vi "UHR-Fleezers Control (host) - 12.2.vi"() -> ()   [LabVIEW 2012] (continued)
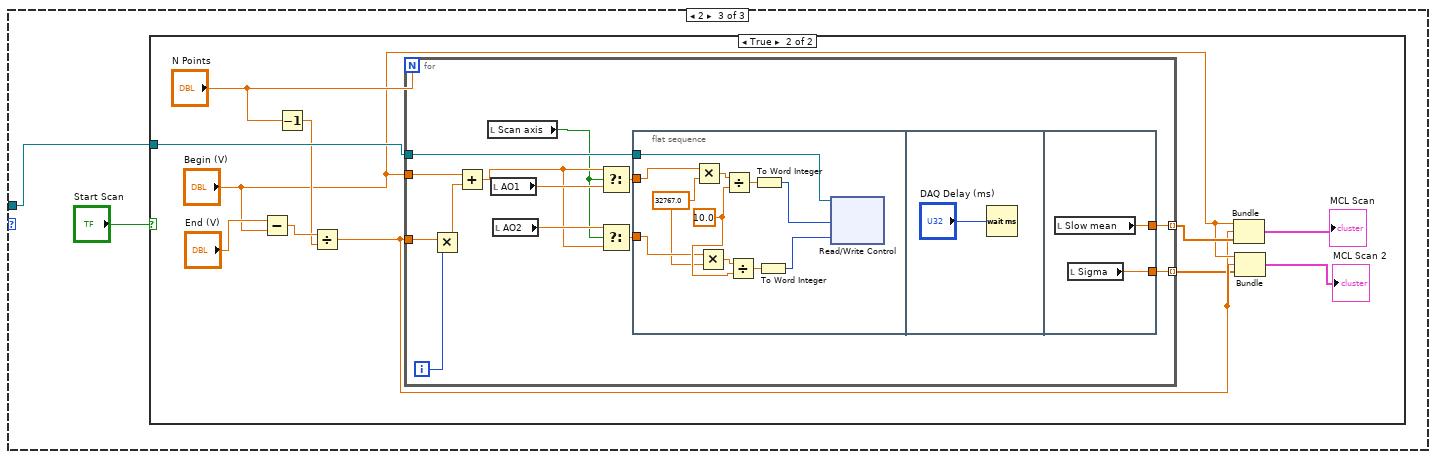
[diagram p3: hidden frame]
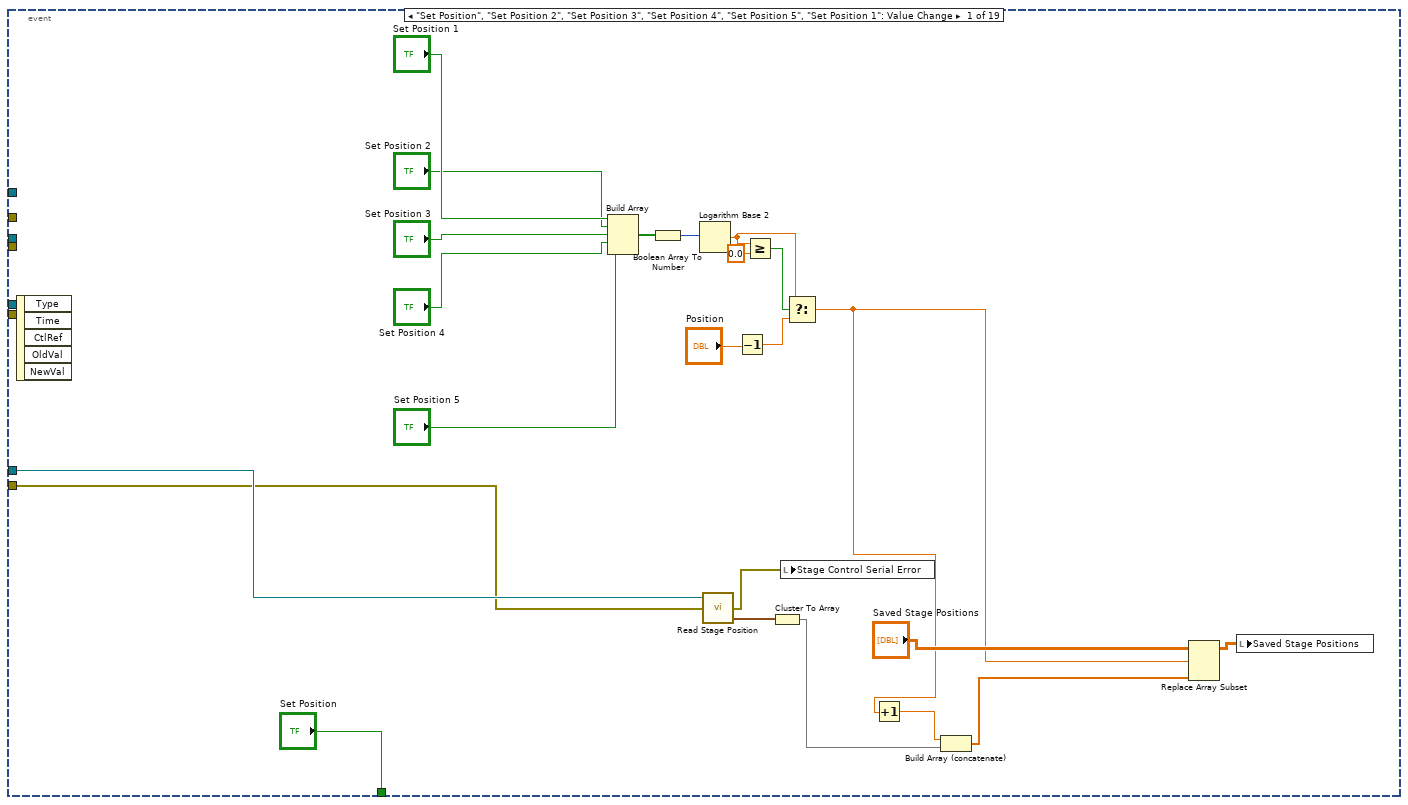
[diagram p6: hidden frame]
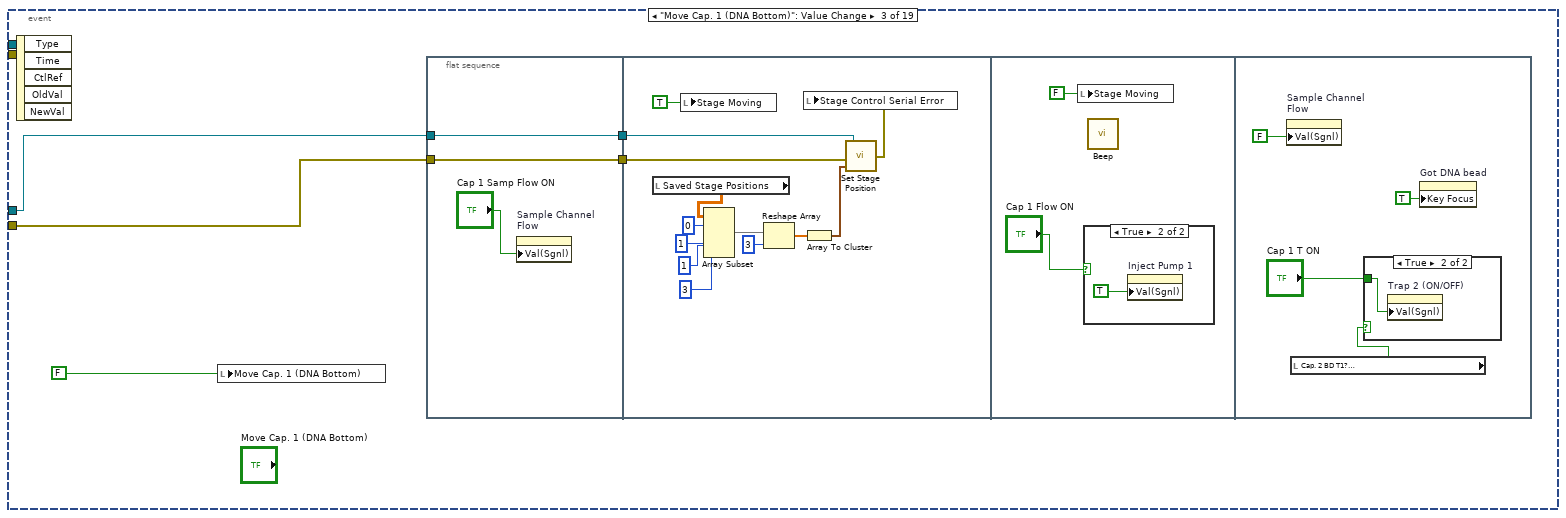
[diagram p7: hidden frame]
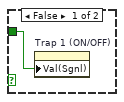
[diagram p9: hidden frame]
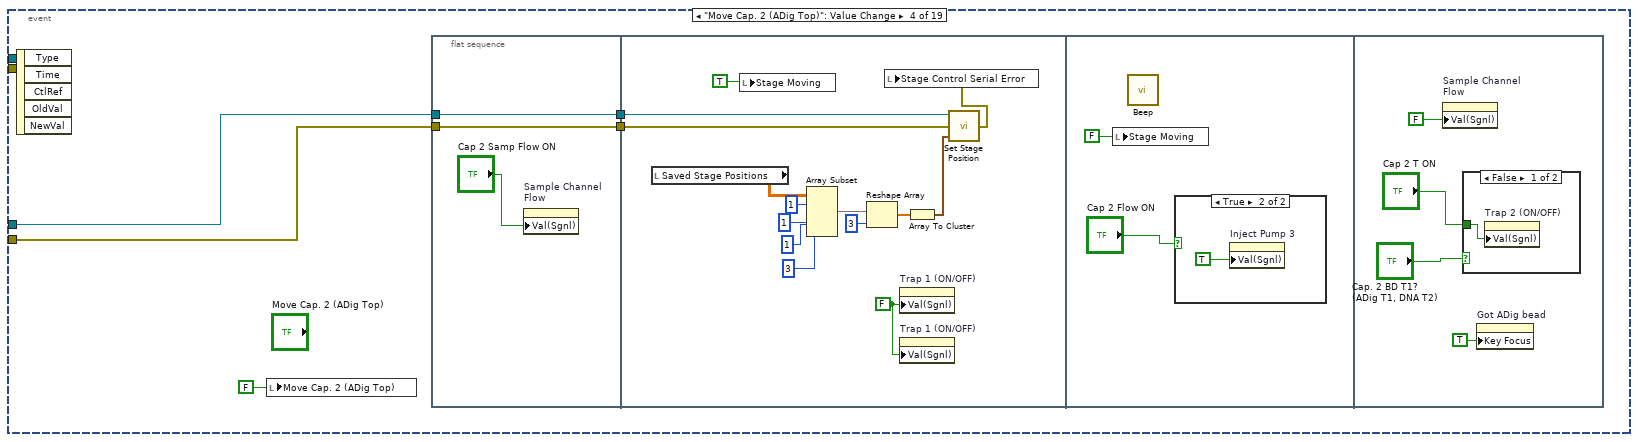
[diagram p10: hidden frame]
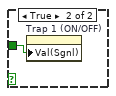
[diagram p12: hidden frame]
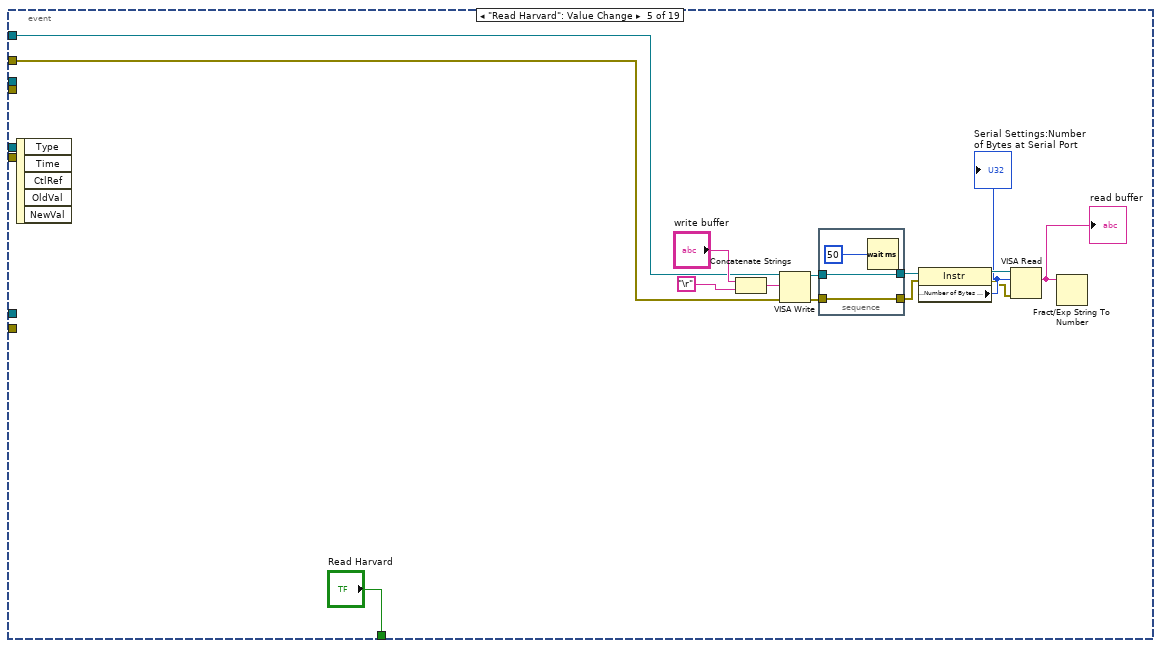
[diagram p13: hidden frame]
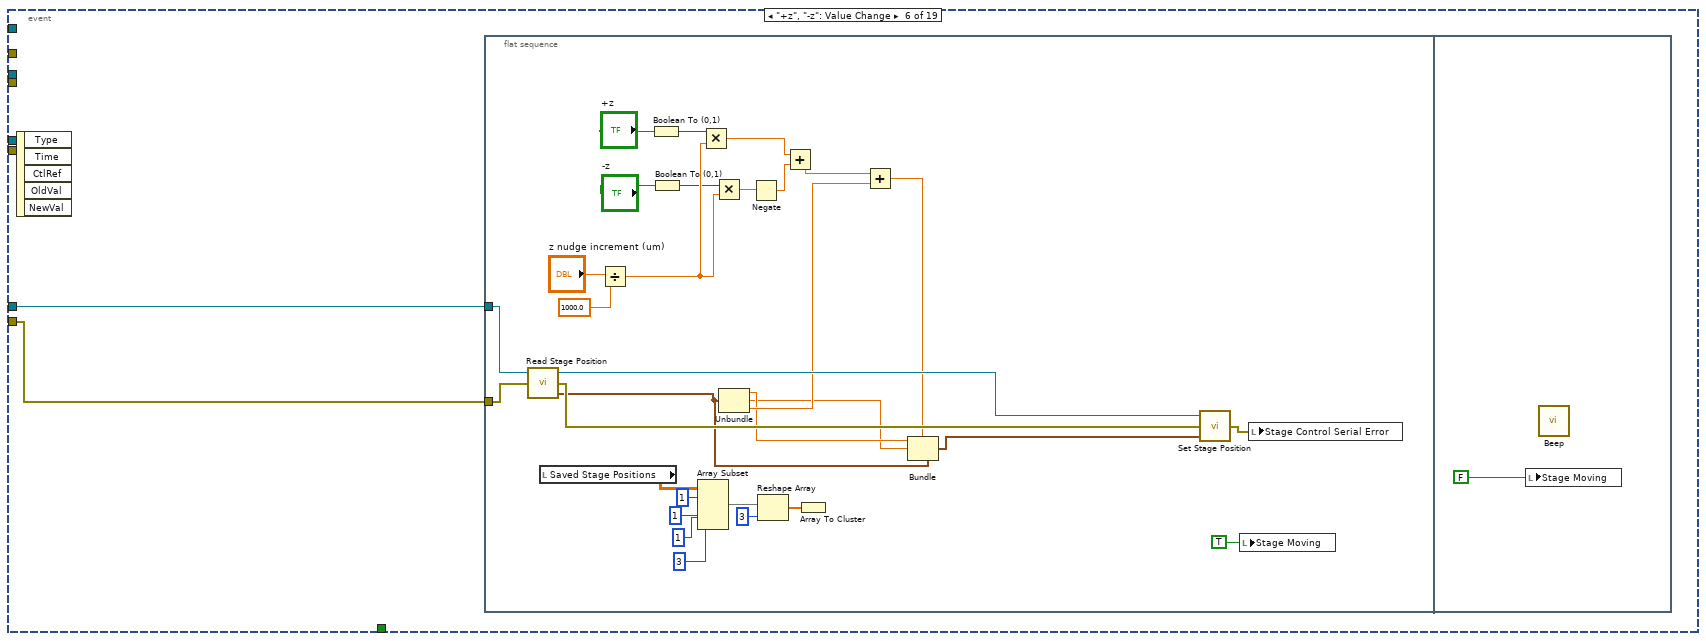
[diagram p14: hidden frame]
                                frame "Image", Default {
                                }
                                frame "Yank" {
                                n2869 = flat-sequence {
                                tunnel: [w4697] -> w4695
                                tunnel: w4694 -> [w4697]
                                tunnel: [w4696] -> w4693
                                tunnel: w4692 -> [w4696]
                                tunnel: w4695 -> [w4703]
                                tunnel: w4693 -> [w4701]
                                frame #0 {
                                n2870 = local read "Yank Delay (s)"() -> (w4700:dbl)
                                n2871 = Multiply(x=w4700, y=1000.0) -> (x*y=w4698:dbl)
                                n2872 = Wait (ms)(milliseconds to wait=w4698) -> ()  [unwired: 1 out]
                                }
                                frame #1 {
                                n2873 = local read "Yank to which?"() -> (w4702:bool)
                                n2874 = case shown="False" w4702 {
                                tunnel: w4703 -> [_ w4731]
                                tunnel: w4701 -> [w4704 _]
                                frame False {
                                n2875 = flat-sequence {
                                tunnel: w4704 -> [w4705]
                                frame #0 {
                                n2876 = property on="Trap Pos FB SP" class="DigNum (strict)"("Val(Sgnl)"=w4705) -> ()  [unwired: 2 in, 2 out]
                                }
                                frame #1 {
                                n2877 = Wait (ms)(milliseconds to wait=u32 700) -> ()  [unwired: 1 out]
                                }
                                frame #2 {
                                n2878 = local read "Action (%)"() -> (w4710:dbl)
                                n2879 = Absolute Value(x=w4710) -> (abs(x)=w4709:dbl)
                                n2880 = Greater?(x=w4709, y=70.0) -> (0:w4707:bool)
                                n2881 = property on="Remove Action Offset" class="Bool (strict)"("Val(Sgnl)"=w4707) -> ()  [unwired: 2 in, 2 out]
                                }
                                frame #3 {
                                n2882 = for {
                                N: 4 -> [_]
                                n2883 = flat-sequence {
                                frame #0 {
                                n2884 = Wait (ms)(milliseconds to wait=u32 500) -> ()  [unwired: 1 out]
                                }
                                frame #1 {
                                n2885 = local read "Action (%)"() -> (w4716:dbl)
                                n2886 = Absolute Value(x=w4716) -> (abs(x)=w4715:dbl)
                                n2887 = Greater?(x=w4715, y=70.0) -> (0:w4713:bool)
                                n2888 = property on="Remove Action Offset" class="Bool (strict)"("Val(Sgnl)"=w4713) -> ()  [unwired: 2 in, 2 out]
                                }
                                }
                                }
                                }
                                frame #4 {
                                n2889 = Wait (ms)(milliseconds to wait=u32 500) -> ()  [unwired: 1 out]
                                }
                                frame #5 {
                                n2890 = local read "Shift confocal"() -> (w4721:bool)
                                n2891 = local read "Mean"() -> (w4724:dbl)
                                n2892 = Greater?(x=w4724, y=11.0) -> (0:w4720:bool)
                                n2893 = Not(x=w4720) -> (.not. x?=w4719:bool)
                                n2894 = And(x=w4720, y=w4721) -> (x .and. y?=w4722:bool)
                                n2895 = And(x=w4719, y=w4721) -> (x .and. y?=w4718:bool)
                                n2896 = case shown="True" w4722 {
                                frame False {
                                }
                                frame True {
                                n2897 = local read "Confocal X 2 (V)"() -> (w4727:dbl)
                                n2898 = local read "Confocal Y 2 (V)"() -> (w4728:dbl)
                                n2899 = property on="AO2" class="Slide (strict)"("Val(Sgnl)"=w4727) -> ()  [unwired: 2 in, 2 out]
                                n2900 = property on="AO1" class="Slide (strict)"("Val(Sgnl)"=w4728) -> ()  [unwired: 2 in, 2 out]
                                }
                                }
                                n2901 = case shown="True" w4718 {
                                frame False {
                                }
                                frame True {
                                n2902 = local read "Confocal Y 1 (V)"() -> (w4726:dbl)
                                n2903 = local read "Confocal X 1 (V)"() -> (w4725:dbl)
                                n2904 = property on="AO1" class="Slide (strict)"("Val(Sgnl)"=w4726) -> ()  [unwired: 2 in, 2 out]
                                n2905 = property on="AO2" class="Slide (strict)"("Val(Sgnl)"=w4725) -> ()  [unwired: 2 in, 2 out]
                                }
                                }
                                }
                                frame #6 {
                                n2906 = Wait (ms)(milliseconds to wait=u32 1500) -> ()  [unwired: 1 out]
                                }
                                frame #7 {
                                n2907 = property on="Rem fb disp offset" class="Bool (strict)"("Val(Sgnl)"=TRUE ("Value (Signaling)")) -> ()  [unwired: 2 in, 2 out]
                                }
                                }
                                }
                                frame True {
                                n2908 = flat-sequence {
                                tunnel: w4731 -> [w4732]
                                frame #0 {
                                n2909 = property on="Trap Delta (MHz)" class="DigNum (strict)"("Val(Sgnl)"=w4732) -> ()  [unwired: 2 in, 2 out]
                                }
                                frame #1 {
                                n2910 = Wait (ms)(milliseconds to wait=u32 500) -> ()  [unwired: 1 out]
                                }
                                frame #2 {
                                n2911 = local read "Shift confocal"() -> (w4738:bool)
                                n2912 = local read "Mean"() -> (w4739:dbl)
                                n2913 = Greater?(x=w4739, y=11.0) -> (0:w4737:bool)
                                n2914 = And(x=w4737, y=w4738) -> (x .and. y?=w4735:bool)
                                n2915 = Not(x=w4737) -> (.not. x?=w4736:bool)
                                n2916 = And(x=w4736, y=w4738) -> (x .and. y?=w4734:bool)
                                n2917 = case shown="True" w4735 {
                                frame False {
                                }
                                frame True {
                                n2918 = local read "Confocal Y 2 (V)"() -> (w4744:dbl)
                                n2919 = local read "Confocal X 2 (V)"() -> (w4743:dbl)
                                n2920 = property on="AO1" class="Slide (strict)"("Val(Sgnl)"=w4744) -> ()  [unwired: 2 in, 2 out]
                                n2921 = property on="AO2" class="Slide (strict)"("Val(Sgnl)"=w4743) -> ()  [unwired: 2 in, 2 out]
                                }
                                }
                                n2922 = case shown="True" w4734 {
                                frame False {
                                }
                                frame True {
                                n2923 = local read "Confocal Y 1 (V)"() -> (w4742:dbl)
                                n2924 = local read "Confocal X 1 (V)"() -> (w4741:dbl)
                                n2925 = property on="AO2" class="Slide (strict)"("Val(Sgnl)"=w4741) -> ()  [unwired: 2 in, 2 out]
                                n2926 = property on="AO1" class="Slide (strict)"("Val(Sgnl)"=w4742) -> ()  [unwired: 2 in, 2 out]
                                }
                                }
                                }
                                }
                                }
                                }
                                }
                                }
                                }
                                }
                                n2927 = local read "Time (s)"() -> (w4679:dbl)
                                n2928 = Subtract(x=w4680, y=w4679) -> (x-y=w4691:dbl)
                                n2929 = Number To Decimal String(number=w4691, width (-)=i16 0) -> (decimal integer string=w4689:string)
                                n2930 = Concatenate Strings(w4689, " s fluorescence event") -> (w4686:string)
                                n2931 = local read "Messages"() -> (w4687:string)
                                n2932 = local write "Duration (s)"(w4691) -> ()
                                n2933 = call "Update messages.vi"("Message to add"=w4686, "Old message string"=w4687) -> ("New message string"=w4685:string)
                                n2934 = local write "Messages"(w4685) -> ()
                                n2935 = call <vilib>:"Beep.vi"() -> ()  [unwired: 12 in]
                                n2936 = local write "Reset Force"(FALSE ("Force Reset")) -> ()
                                n2937 = local write "Fl. High"(TRUE ("Fl. High")) -> ()
                                n2938 = local write "Waiting"(TRUE ("Waiting")) -> ()
                                }
                                }
                                n2939 = node-c288() -> ()  [unwired: 1 in, 1 out]
                                }
                                n2940 = node-c288(w4658) -> ()  [unwired: 1 out]
                                }
                              }
                            }
                          }
                          n2941 = local read "Trap Delta (MHz)"() -> (w4570:dbl)
                          n2942 = local read "Trap Pos FB SP"() -> (w4568:fxp<+/-,16,1>)
                        }
                      }
                    }
                    frame True {
                      n2943 = flat-sequence {
                        tunnel: w4755 -> [w4765]
                        tunnel: [w4765] -> w4759
                        tunnel: w4758 -> [w4764]
                        tunnel: [w4764] -> w4757
                        tunnel: [w4763] -> w4756
                        tunnel: w4754 -> [w4762]
                        tunnel: [w4761] -> w4753
                        tunnel: w4750 -> [w4760]
                        tunnel: [w4760] -> w4749
                        tunnel: w4759 -> [w4835]
                        tunnel: w4757 -> [w4834]
                        tunnel: w4756 -> [w4833]
                        tunnel: w4753 -> [w4832]
                        tunnel: w4749 -> [w4831]
                        tunnel: [w4832] -> w4752
                        frame #0 {
                          n2944 = call <vilib>:"Beep.vi"() -> ()  [unwired: 3 in, 9 out]
                          n2945 = local write "Waiting"(FALSE ("Waiting")) -> ()
                          n2946 = Increment(x=w4762) -> (x+1=w4761:u8)
                          n2947 = case shown="\"Yank\"" w4764 {
                            tunnel: w4761 -> [_ _ w4771]
                            frame "Image" {
                              n2948 = property on="Confocal Image" class="Bool (strict)"("Val(Sgnl)"=TRUE ("Value (Signaling)")) -> ()  [unwired: 2 in, 2 out]
                            }
                            frame "Alarm", Default {
                            }
                            frame "Yank" {
                              n2949 = flat-sequence {
                                tunnel: w4771 -> [w4774]
                                tunnel: [w4773] -> w4770
                                tunnel: ["N Array El"] -> w4769
                                tunnel: w4770 -> [w4788]
                                tunnel: w4769 -> [w4784]
                                frame #0 {
                                n2950 = Multiply(x="Yank Delay (s)", y=1000.0) -> (x*y=w4777:dbl)
                                n2951 = Quotient & Remainder(x=w4774, y="N Array El") -> (x-y*floor(x/y)=w4773:u8)  [unwired: 1 out]
                                n2952 = Wait (ms)(milliseconds to wait=w4777) -> ()  [unwired: 1 out]
                                }
                                frame #1 {
                                n2953 = Random Number (0-1)() -> (number: 0 to 1=w4785:dbl)
                                n2954 = Multiply(x=w4784, y=w4785) -> (x*y=w4783:dbl)
                                n2955 = Round Toward -Infinity(1:w4783) -> (0:w4782:dbl)
                                n2956 = Select(t=w4782, s="Random Choice", f=w4788) -> (s? t:f=w4786:dbl)
                                n2957 = Select(t="Yank to Trap Delta (MHz)", s="Yank to which?", f="Yank to SP") -> (s? t:f=w4779:dbl[])
                                n2958 = Index Array(array=w4779, index=w4786) -> (element=w4789:dbl)
                                n2959 = case shown="False" "Yank to which?" {
                                tunnel: w4789 -> [w4790 w4816]
                                frame False {
                                n2960 = flat-sequence {
                                tunnel: w4790 -> [w4791]
                                frame #0 {
                                n2961 = property on="Trap Pos FB SP" class="DigNum (strict)"("Val(Sgnl)"=w4791) -> ()  [unwired: 2 in, 2 out]
                                }
                                frame #1 {
                                n2962 = Wait (ms)(milliseconds to wait=u32 700) -> ()  [unwired: 1 out]
                                }
                                frame #2 {
                                n2963 = local read "Action (%)"() -> (w4796:dbl)
                                n2964 = Absolute Value(x=w4796) -> (abs(x)=w4795:dbl)
                                n2965 = Greater?(x=w4795, y=70.0) -> (0:w4793:bool)
                                n2966 = property on="Remove Action Offset" class="Bool (strict)"("Val(Sgnl)"=w4793) -> ()  [unwired: 2 in, 2 out]
                                }
                                frame #3 {
                                n2967 = for {
                                N: 4 -> [_]
                                n2968 = flat-sequence {
                                frame #0 {
                                n2969 = Wait (ms)(milliseconds to wait=u32 500) -> ()  [unwired: 1 out]
                                }
                                frame #1 {
                                n2970 = local read "Action (%)"() -> (w4802:dbl)
                                n2971 = Absolute Value(x=w4802) -> (abs(x)=w4801:dbl)
                                n2972 = Greater?(x=w4801, y=70.0) -> (0:w4799:bool)
                                n2973 = property on="Remove Action Offset" class="Bool (strict)"("Val(Sgnl)"=w4799) -> ()  [unwired: 2 in, 2 out]
                                }
                                }
                                }
                                }
                                frame #4 {
                                n2974 = local read "Shift confocal"() -> (w4806:bool)
                                n2975 = local read "Mean"() -> (w4809:dbl)
                                n2976 = Greater?(x=w4809, y=11.0) -> (0:w4805:bool)
                                n2977 = Not(x=w4805) -> (.not. x?=w4804:bool)
                                n2978 = And(x=w4804, y=w4806) -> (x .and. y?=w4803:bool)
                                n2979 = And(x=w4805, y=w4806) -> (x .and. y?=w4807:bool)
                                n2980 = case shown="True" w4807 {
                                frame False {
                                }
                                frame True {
                                n2981 = local read "Confocal X 2 (V)"() -> (w4812:dbl)
                                n2982 = local read "Confocal Y 2 (V)"() -> (w4813:dbl)
                                n2983 = property on="AO2" class="Slide (strict)"("Val(Sgnl)"=w4812) -> ()  [unwired: 2 in, 2 out]
                                n2984 = property on="AO1" class="Slide (strict)"("Val(Sgnl)"=w4813) -> ()  [unwired: 2 in, 2 out]
                                }
                                }
                                n2985 = case shown="True" w4803 {
                                frame False {
                                }
                                frame True {
                                n2986 = local read "Confocal X 1 (V)"() -> (w4810:dbl)
                                n2987 = local read "Confocal Y 1 (V)"() -> (w4811:dbl)
                                n2988 = property on="AO1" class="Slide (strict)"("Val(Sgnl)"=w4811) -> ()  [unwired: 2 in, 2 out]
                                n2989 = property on="AO2" class="Slide (strict)"("Val(Sgnl)"=w4810) -> ()  [unwired: 2 in, 2 out]
                                }
                                }
                                }
                                frame #5 {
                                n2990 = Wait (ms)(milliseconds to wait=u32 1500) -> ()  [unwired: 1 out]
                                }
                                frame #6 {
                                n2991 = property on="Rem fb disp offset" class="Bool (strict)"("Val(Sgnl)"=TRUE ("Value (Signaling)")) -> ()  [unwired: 2 in, 2 out]
                                }
                                }
                                }
                                frame True {
                                n2992 = flat-sequence {
                                tunnel: w4816 -> [w4817]
                                frame #0 {
                                n2993 = property on="Trap Delta (MHz)" class="DigNum (strict)"("Val(Sgnl)"=w4817) -> ()  [unwired: 2 in, 2 out]
                                }
                                frame #1 {
                                n2994 = Wait (ms)(milliseconds to wait=u32 500) -> ()  [unwired: 1 out]
                                }
                                frame #2 {
                                n2995 = local read "Shift confocal"() -> (w4821:bool)
                                n2996 = local read "Mean"() -> (w4819:dbl)
                                n2997 = Greater?(x=w4819, y=11.0) -> (0:w4822:bool)
                                n2998 = Not(x=w4822) -> (.not. x?=w4823:bool)
                                n2999 = And(x=w4823, y=w4821) -> (x .and. y?=w4825:bool)
                                n3000 = And(x=w4822, y=w4821) -> (x .and. y?=w4824:bool)
                                n3001 = case shown="True" w4824 {
                                frame False {
                                }
                                frame True {
                                n3002 = local read "Confocal Y 2 (V)"() -> (w4829:dbl)
                                n3003 = local read "Confocal X 2 (V)"() -> (w4828:dbl)
                                n3004 = property on="AO1" class="Slide (strict)"("Val(Sgnl)"=w4829) -> ()  [unwired: 2 in, 2 out]
                                n3005 = property on="AO2" class="Slide (strict)"("Val(Sgnl)"=w4828) -> ()  [unwired: 2 in, 2 out]
                                }
                                }
                                n3006 = case shown="True" w4825 {
                                frame False {
                                }
                                frame True {
                                n3007 = local read "Confocal X 1 (V)"() -> (w4826:dbl)
                                n3008 = local read "Confocal Y 1 (V)"() -> (w4827:dbl)
                                n3009 = property on="AO2" class="Slide (strict)"("Val(Sgnl)"=w4826) -> ()  [unwired: 2 in, 2 out]
                                n3010 = property on="AO1" class="Slide (strict)"("Val(Sgnl)"=w4827) -> ()  [unwired: 2 in, 2 out]
                                }
                                }
                                }
                                }
                                }
                                }
                                }
                              }
                            }
                          }
                          n3011 = local read "Time (s)"() -> (w4763:dbl)
                          "Fl. High" <- TRUE ("Yanking")
                        }
                        frame #1 {
                          n3012 = local read "Auto F Reset"() -> (w4830:bool)
                          n3013 = case shown="True" w4830 {
                            tunnel: w4835 -> [_ w4839]
                            tunnel: w4834 -> [_ w4838]
                            tunnel: w4833 -> [_ w4837]
                            tunnel: w4831 -> [_ w4836]
                            frame False {
                            }
                            frame True {
                              n3014 = node-c288() -> (w4841:T21)  [unwired: 4 out]
                              n3015 = timed-loop {
                                timing: w4841 -> [_]
                                timing-out: [_] -> w4840
                                tunnel: w4839 -> [w4859]
                                tunnel: w4838 -> [w4858]
                                tunnel: w4837 -> [w4857]
                                tunnel: w4836 -> [w4856]
                                stop <- w4842 stop-if-true
                                n3016 = node-c288() -> ()  [unwired: 2 out]
                                n3017 = local read "Fl. Delta Thresh. (kHz)"() -> (w4850:dbl)
                                n3018 = local read "Fl. Triggered..."() -> (w4855:bool)
                                n3019 = local read "Delta Fl. 1"() -> (w4846:dbl)
                                n3020 = local read "Delta Fl. 2"() -> (w4844:dbl)
                                n3021 = local read "Stop All"() -> (w4853:bool)
                                n3022 = local read "APD to Watch"() -> (w4845:bool)
                                n3023 = Select(t=w4846, s=w4845, f=w4844) -> (s? t:f=w4843:dbl)
                                n3024 = Not(x=w4855) -> (.not. x?=w4854:bool)
                                n3025 = Multiply(x=w4850, y=1000.0) -> (x*y=w4849:dbl)
                                n3026 = Negate(x=w4849) -> (-x=w4848:dbl)
                                n3027 = Less?(x=w4843, y=w4848) -> (x < y?=w4852:bool)
                                n3028 = Compound Arithmetic op=OR(w4852, w4853, w4854, "Reset Force") -> (w4842:bool)
                                n3029 = case shown="True" w4842 {
                                tunnel: w4859 -> [_ w4874]
                                tunnel: w4858 -> [_ w4873]
                                tunnel: w4857 -> [_ w4863]
                                tunnel: w4856 -> [_ w4865]
                                frame False {
                                }
                                frame True {
                                n3030 = local read "Time (s)"() -> (w4864:dbl)
                                n3031 = case shown="\"Yank\"" w4873 {
                                tunnel: w4874 -> [_ w4877]
                                tunnel: w4865 -> [_ w4875]
                                frame "Image", Default {
                                }
                                frame "Yank" {
                                n3032 = flat-sequence {
                                tunnel: [w4883] -> w4878
                                tunnel: w4877 -> [w4883]
                                tunnel: [w4879] -> w4876
                                tunnel: w4875 -> [w4879]
                                tunnel: w4878 -> [w4886]
                                tunnel: w4876 -> [w4884]
                                frame #0 {
                                n3033 = local read "Yank Delay (s)"() -> (w4882:dbl)
                                n3034 = Multiply(x=w4882, y=1000.0) -> (x*y=w4880:dbl)
                                n3035 = Wait (ms)(milliseconds to wait=w4880) -> ()  [unwired: 1 out]
                                }
                                frame #1 {
                                n3036 = local read "Yank to which?"() -> (w4885:bool)
                                n3037 = case shown="False" w4885 {
                                tunnel: w4886 -> [_ w4913]
                                tunnel: w4884 -> [w4887 _]
                                frame False {
                                n3038 = flat-sequence {
                                tunnel: w4887 -> [w4888]
                                frame #0 {
                                n3039 = property on="Trap Pos FB SP" class="DigNum (strict)"("Val(Sgnl)"=w4888) -> ()  [unwired: 2 in, 2 out]
                                }
                                frame #1 {
                                n3040 = Wait (ms)(milliseconds to wait=u32 700) -> ()  [unwired: 1 out]
                                }
                                frame #2 {
                                n3041 = local read "Action (%)"() -> (w4893:dbl)
                                n3042 = Absolute Value(x=w4893) -> (abs(x)=w4892:dbl)
                                n3043 = Greater?(x=w4892, y=70.0) -> (0:w4890:bool)
                                n3044 = property on="Remove Action Offset" class="Bool (strict)"("Val(Sgnl)"=w4890) -> ()  [unwired: 2 in, 2 out]
                                }
                                frame #3 {
                                n3045 = for {
                                N: 4 -> [_]
                                n3046 = flat-sequence {
                                frame #0 {
                                n3047 = Wait (ms)(milliseconds to wait=u32 500) -> ()  [unwired: 1 out]
                                }
                                frame #1 {
                                n3048 = local read "Action (%)"() -> (w4899:dbl)
                                n3049 = Absolute Value(x=w4899) -> (abs(x)=w4898:dbl)
                                n3050 = Greater?(x=w4898, y=70.0) -> (0:w4896:bool)
                                n3051 = property on="Remove Action Offset" class="Bool (strict)"("Val(Sgnl)"=w4896) -> ()  [unwired: 2 in, 2 out]
                                }
                                }
                                }
                                }
                                frame #4 {
                                n3052 = local read "Shift confocal"() -> (w4904:bool)
                                n3053 = local read "Mean"() -> (w4906:dbl)
                                n3054 = Greater?(x=w4906, y=11.0) -> (0:w4903:bool)
                                n3055 = Not(x=w4903) -> (.not. x?=w4902:bool)
                                n3056 = And(x=w4903, y=w4904) -> (x .and. y?=w4901:bool)
                                n3057 = And(x=w4902, y=w4904) -> (x .and. y?=w4900:bool)
                                n3058 = case shown="True" w4901 {
                                frame False {
                                }
                                frame True {
                                n3059 = local read "Confocal Y 2 (V)"() -> (w4910:dbl)
                                n3060 = local read "Confocal X 2 (V)"() -> (w4909:dbl)
                                n3061 = property on="AO2" class="Slide (strict)"("Val(Sgnl)"=w4909) -> ()  [unwired: 2 in, 2 out]
                                n3062 = property on="AO1" class="Slide (strict)"("Val(Sgnl)"=w4910) -> ()  [unwired: 2 in, 2 out]
                                }
                                }
                                n3063 = case shown="True" w4900 {
                                frame False {
                                }
                                frame True {
                                n3064 = local read "Confocal X 1 (V)"() -> (w4907:dbl)
                                n3065 = local read "Confocal Y 1 (V)"() -> (w4908:dbl)
                                n3066 = property on="AO1" class="Slide (strict)"("Val(Sgnl)"=w4908) -> ()  [unwired: 2 in, 2 out]
                                n3067 = property on="AO2" class="Slide (strict)"("Val(Sgnl)"=w4907) -> ()  [unwired: 2 in, 2 out]
                                }
                                }
                                }
                                frame #5 {
                                n3068 = Wait (ms)(milliseconds to wait=u32 1500) -> ()  [unwired: 1 out]
                                }
                                frame #6 {
                                n3069 = property on="Rem fb disp offset" class="Bool (strict)"("Val(Sgnl)"=TRUE ("Value (Signaling)")) -> ()  [unwired: 2 in, 2 out]
                                }
                                }
                                }
                                frame True {
                                n3070 = flat-sequence {
                                tunnel: w4913 -> [w4914]
                                frame #0 {
                                n3071 = property on="Trap Delta (MHz)" class="DigNum (strict)"("Val(Sgnl)"=w4914) -> ()  [unwired: 2 in, 2 out]
                                }
                                frame #1 {
                                n3072 = Wait (ms)(milliseconds to wait=u32 500) -> ()  [unwired: 1 out]
                                }
                                frame #2 {
                                n3073 = local read "Shift confocal"() -> (w4920:bool)
                                n3074 = local read "Mean"() -> (w4922:dbl)
                                n3075 = Greater?(x=w4922, y=11.0) -> (0:w4919:bool)
                                n3076 = Not(x=w4919) -> (.not. x?=w4918:bool)
                                n3077 = And(x=w4919, y=w4920) -> (x .and. y?=w4917:bool)
                                n3078 = And(x=w4918, y=w4920) -> (x .and. y?=w4916:bool)
                                n3079 = case shown="True" w4917 {
                                frame False {
                                }
                                frame True {
                                n3080 = local read "Confocal Y 2 (V)"() -> (w4926:dbl)
                                n3081 = local read "Confocal X 2 (V)"() -> (w4925:dbl)
                                n3082 = property on="AO2" class="Slide (strict)"("Val(Sgnl)"=w4925) -> ()  [unwired: 2 in, 2 out]
                                n3083 = property on="AO1" class="Slide (strict)"("Val(Sgnl)"=w4926) -> ()  [unwired: 2 in, 2 out]
                                }
                                }
                                n3084 = case shown="True" w4916 {
                                frame False {
                                }
                                frame True {
                                n3085 = local read "Confocal Y 1 (V)"() -> (w4924:dbl)
                                n3086 = local read "Confocal X 1 (V)"() -> (w4923:dbl)
                                n3087 = property on="AO2" class="Slide (strict)"("Val(Sgnl)"=w4923) -> ()  [unwired: 2 in, 2 out]
                                n3088 = property on="AO1" class="Slide (strict)"("Val(Sgnl)"=w4924) -> ()  [unwired: 2 in, 2 out]
                                }
                                }
                                }
                                }
                                }
                                }
                                }
                                }
                                }
                                }
                                n3089 = local read "Messages"() -> (w4872:string)
                                n3090 = Subtract(x=w4864, y=w4863) -> (x-y=w4870:dbl)
                                "Duration (s)" <- w4870
                                n3091 = Number To Decimal String(number=w4870, width (-)=i16 0) -> (decimal integer string=w4868:string)
                                n3092 = Concatenate Strings(w4868, " s fluorescence event." ("string")) -> (w4866:string)
                                n3093 = call "Update messages.vi"("Message to add"=w4866, "Old message string"=w4872) -> ("New message string"=w4871:string)
                                n3094 = local write "Reset Force"(FALSE ("Reset Force")) -> ()
                                n3095 = local write "Waiting"(TRUE ("Waiting")) -> ()
                                n3096 = local write "Messages"(w4871) -> ()
                                n3097 = local write "Fl. High"(FALSE ("Fl. High")) -> ()
                                n3098 = call <vilib>:"Beep.vi"() -> ()  [unwired: 3 in, 9 out]
                                }
                                }
                                n3099 = node-c288() -> ()  [unwired: 2 out]
                              }
                              n3100 = node-c288(w4840) -> ()  [unwired: 1 out]
                            }
                          }
                        }
                      }
                      n3101 = local read "Trap Delta (MHz)"() -> (w4755:dbl)
                      n3102 = local read "Trap Pos FB SP"() -> (w4750:fxp<+/-,16,1>)
                    }
                  }
                }
                frame #1 {
                  n3103 = local read "Stop All"() -> (w4936:bool)
                  n3104 = local read "Fl. Triggered..."() -> (w4934:bool)
                  n3105 = Not(x=w4934) -> (.not. x?=w4935:bool)
                  n3106 = Or(x=w4935, y=w4936) -> (x .or. y?=w4933:bool)
                }
              }
              n3107 = case shown="True" w4527 {
                frame False {
                }
                frame True {
                  n3108 = local read "Confocal Y 1 (V)"() -> (w4537:dbl)
                  n3109 = local read "Confocal X 1 (V)"() -> (w4536:dbl)
                  n3110 = property on="AO2" class="Slide (strict)"("Val(Sgnl)"=w4536) -> ()  [unwired: 2 in, 2 out]
                  n3111 = property on="AO1" class="Slide (strict)"("Val(Sgnl)"=w4537) -> ()  [unwired: 2 in, 2 out]
                }
              }
              n3112 = case shown="True" w4527 {
                frame False {
                }
                frame True {
                  w4535 = FALSE ("Fl. High")
                  n3113 = local write "Waiting"(w4535) -> ()
                  n3114 = local write "Fl. High"(w4535) -> ()
                }
              }
              n3115 = node-c288() -> ()  [unwired: 2 out]
            }
            n3116 = node-c288(w4525) -> ()  [unwired: 1 out]
          }
        }
      }
      event "Stop All": Value Change {
        n3117 = event-data() -> ()  [unwired: 7 out]
        n3118 = local read "Stop All"() -> (w4941:bool)
      }
    }
    n3119 = node-c288() -> ()  [unwired: 2 out]
  }
  n3120 = node-c288(w1) -> ()  [unwired: 1 out]
  n3121 = node-c288(w136) -> ()  [unwired: 1 out]
  n3122 = node-c288(w138) -> ()  [unwired: 1 out]
  n3123 = node-c288(w123) -> ()  [unwired: 1 out]
  n3124 = property on="Saved trap pos" class="WFGraph (strict)"("Visible"=FALSE) -> ()  [unwired: 2 in, 2 out]
  n3125 = property on="Trap Delta Graph" class="WFGraph (strict)"("Visible"=TRUE) -> ()  [unwired: 2 in, 2 out]
  n3126 = local write "Trap pos"(FALSE ("Trap pos")) -> ()
  n3127 = local write "Offset (nm)"(0.0 ("Offset (nm)")) -> ()
  n3128 = local write "Bead Mean (nm)"(0.0 ("Bead Mean (nm)")) -> ()
  n3129 = disable-structure shown="Disabled" {
    disable-tunnel: w127 -> [w4943 _]
    disable-tunnel: w126 -> [w4942 _]
    frame Disabled {
      n3130 = VISA Close(VISA resource name=w4943, error in (no error)=w4942) -> (error out=w4944:errorcluster)
      n3131 = call <vilib>:"Simple Error Handler.vi"("error in (no error)"=w4944) -> ()  [unwired: 1 in, 8 out]
    }
    frame Enabled {
    }
  }
  n3132 = node-c288(w212) -> ()  [unwired: 1 out]
  n3133 = node-c288(w134) -> ()  [unwired: 1 out]
  n3134 = flat-sequence {
    tunnel: w303 -> [w4948]
    tunnel: w305 -> [w4949]
    tunnel: [w4947] -> w284
    tunnel: [w4946] -> w283
    tunnel: w268 -> [_]
    tunnel: w220 -> [_]
    tunnel: w140 -> [_]
    tunnel: w284 -> [w4950]
    tunnel: w283 -> [w4951]
    frame #0 {
      w4945 = FALSE ("AI to FIFO")
      n3135 = xnode "Read/Write Control"("FPGA VI Reference In"=w4949, "error in"=w4948, "AI to FIFO"=w4945, "APD to FIFO"=w4945) -> ("FPGA VI Reference Out"=w4947:T19, "error out"=w4946:errorcluster)
    }
    frame #1 {
      n3136 = xnode "Close FPGA VI Reference"("FPGA VI Reference In"=w4950, "error in"=w4951) -> ("error out"=→"error out":errorcluster)
    }
  }
